vi "Connect.vi"(8 "error in":errorcluster, 11 "TCP in":refnum<class "TCP.lvclass">) -> (0 "error out":errorcluster, 3 "TCP out":refnum<class "TCP.lvclass">)   [LabVIEW 2021, in "TCP.lvclass"]
uses:
  TCP.lvclass
  controls/INI FGV States.ctl
  TCP.lvclass/TCP.ctl
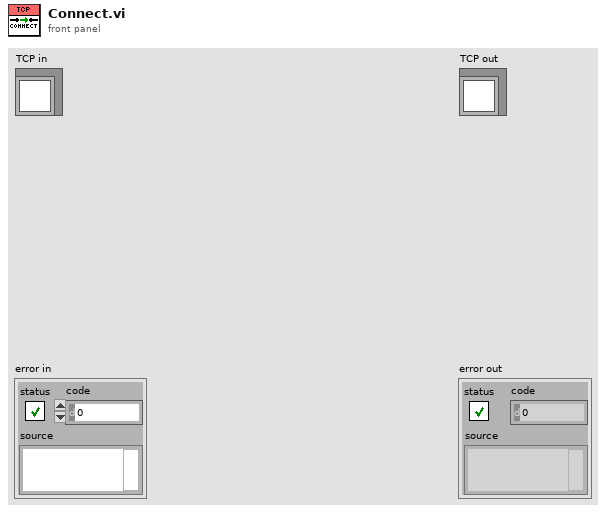
[diagram p1: front panel]
types:
  T1 = typedef "INI FGV States.ctl" = enum16{"Open File", "Read Config", "Write Config", "Close File"}
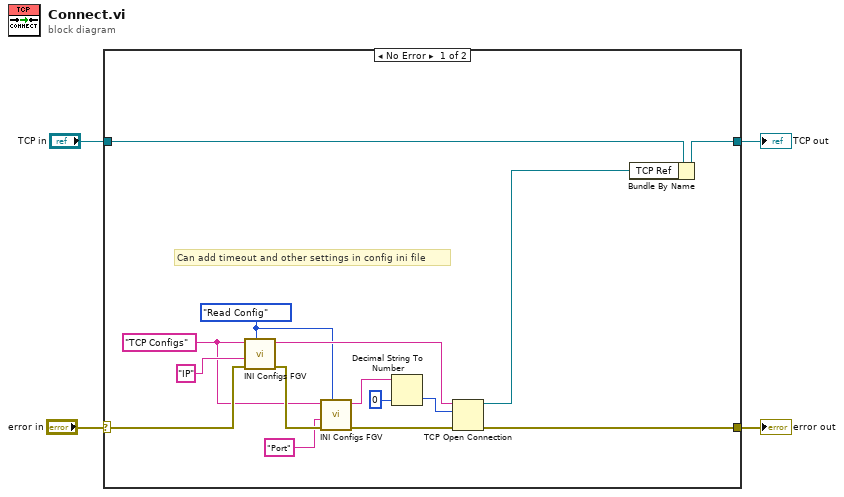
[diagram p0: block diagram]
diagram:
  n1 = case shown="No Error" "error in" {
    selector: "error in" -> [w19 w20]
    tunnel: "TCP in" -> [w18 w21]
    tunnel: [w9 w21] -> w2
    tunnel: [w17 w20] -> w1
    frame No Error {
      w13 = "TCP Configs" ("section")
      w11 = INI_FGV_States."Read Config" ("State")
      # "Can add timeout and other settings in config ini file"
      n2 = call "INI Configs FGV.vi"("State"=w11, "error in"=w19, "key"="IP", "section"=w13) -> ("error out"=w14:errorcluster, "value"=w15:string)  [unwired: 6 in]
      n3 = call "INI Configs FGV.vi"("State"=w11, "error in"=w14, "key"="Port", "section"=w13) -> ("error out"=w10:errorcluster, "value"=w7:string)  [unwired: 6 in]
      n4 = Decimal String To Number(string=w7, default (0L)=u16 0 ("remote port or service name")) -> (number=w5:u16)  [unwired: 1 in, 1 out]
      n5 = TCP Open Connection(address=w15, remote port or service name=w5, error in (no error)=w10) -> (connection ID=w8:refnum<k5>, error out=w17:errorcluster)  [unwired: 2 in]
      n6 = Bundle By Name(cluster=w18, "TCP Ref"=w8) -> (w9:refnum<class "TCP.lvclass">)
    }
    frame Error {
    }
  }
  "error out" <- w1
  "TCP out" <- w2
